vi "GetContent.vi"(8 "Error In":errorcluster, 11 "reference in":refnum<class "BoldDecorator.lvclass">) -> (0 "Error Out":errorcluster, 2 "Content":string, 3 "reference out":refnum<class "BoldDecorator.lvclass">)   [LabVIEW 2024, in "BoldDecorator.lvclass"]
uses:
  BoldDecorator.lvclass
  IText/IText.lvclass
  BoldDecorator.lvclass/BoldDecorator.ctl
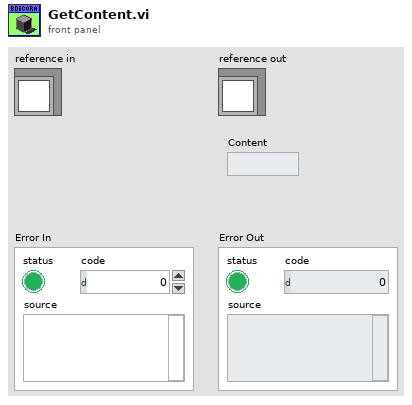
[diagram p1: front panel]
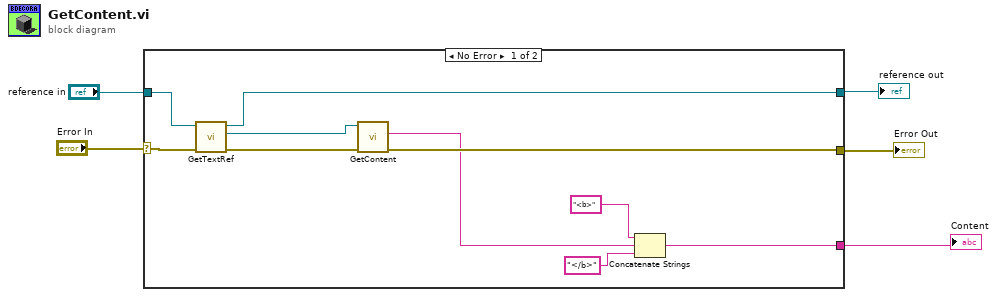
[diagram p0: block diagram]
diagram:
  n1 = case shown="No Error" "Error In" {
    selector: "Error In" -> [w15 w16]
    tunnel: [w10 w16] -> w4
    tunnel: "reference in" -> [w13 w17]
    tunnel: [w12 w17] -> w2
    tunnel: [w11 _] -> w1
    frame No Error {
      n2 = call-dynamic "GetTextRef.vi"("Error In"=w15, "reference in"=w13) -> ("Error Out"=w14:errorcluster, "TextRef"=w9:refnum<class "IText.lvclass">, "reference out"=w12:refnum<class "BoldDecorator.lvclass">)  [unwired: 7 in]
      n3 = call-dynamic "GetContent.vi"("Error In"=w14, "object in"=w9) -> ("Error Out"=w10:errorcluster, "Content"=w8:string)  [unwired: 7 in, 1 out]
      n4 = Concatenate Strings("<b>" ("string"), w8, "</b>" ("string")) -> (w11:string)
    }
    frame Error {
    }
  }
  "Error Out" <- w4
  "reference out" <- w2
  "Content" <- w1
